vi "MS SQL_Count_RFID_STN10.vi"(8 "error in (no error)":errorcluster, 11 "Ref in":T1={"MS SQL Connection"=refnum, "UDL File"=path "", "Time"="", "DCODE"="", "WIP+1"=0, "MC No?"=0, "POKAYOKE?"=FALSE, "Expected Result"="", "Result [Status]"="", "Clock"=0.0, "RFID"="", "WIP Queue"=refnum, "TS Parameter"={"ProfitCenterCode"="", "LineCode"="", "WorkOrderNumber"="", "Model"="", "Model_with_Prefix"="", "VendorCode"="", "SetParameterDateCode"="", "PokaYoke"=0, "Target"=1, "Live_DateCode"="", "CustomerPartNumber"="", "Hand"="", "sBarcode"=FALSE, "FCA"=0, "Ent_Stamp"=timestamp(0 s since 1904-01-01), "STS_CD"=0.0}, "Data_Queue"=[], "RFID Serial No."=""} {"TS Parameter"."FCA" format="%01d"; "TS Parameter"."Target" min=1 max=100000; "TS Parameter"."PokaYoke" min=0 max=1}) -> (0 "error out":errorcluster, 1 "Count":i32 format="%02d", 2 "Count[s]":string, 3 "Ref Out":T1={"MS SQL Connection"=refnum, "UDL File"=path "", "Time"="", "DCODE"="", "WIP+1"=0, "MC No?"=0, "POKAYOKE?"=FALSE, "Expected Result"="", "Result [Status]"="", "Clock"=0.0, "RFID"="", "WIP Queue"=refnum, "TS Parameter"={"ProfitCenterCode"="", "LineCode"="", "WorkOrderNumber"="", "Model"="", "Model_with_Prefix"="", "VendorCode"="", "SetParameterDateCode"="", "PokaYoke"=0, "Target"=1, "Live_DateCode"="", "CustomerPartNumber"="", "Hand"="", "sBarcode"=FALSE, "FCA"=0, "Ent_Stamp"=timestamp(0 s since 1904-01-01), "STS_CD"=0.0}, "Data_Queue"=[], "RFID Serial No."=""} {"TS Parameter"."FCA" format="%01d"; "TS Parameter"."Target" min=1 max=100000; "TS Parameter"."PokaYoke" min=0 max=1}, 4 "resulting string":string)   [LabVIEW 2020]
uses:
  Controls/TD SQL.ctl
  <vilib>/addons/database/Connection.llb/Conn ObjectReference.ctl
  Controls/WIP_State.ctl
  Controls/TS_Parameter.ctl
  <vilib>/addons/database/Connection.llb/Conn Execute.vi
  <vilib>/addons/database/Recordset.llb/Rec Fetch Recordset Data (R).vi
  <vilib>/addons/database/Recordset.llb/Rec Destroy - Connection.vi
  <vilib>/addons/database/NI_Database_API.lvlib
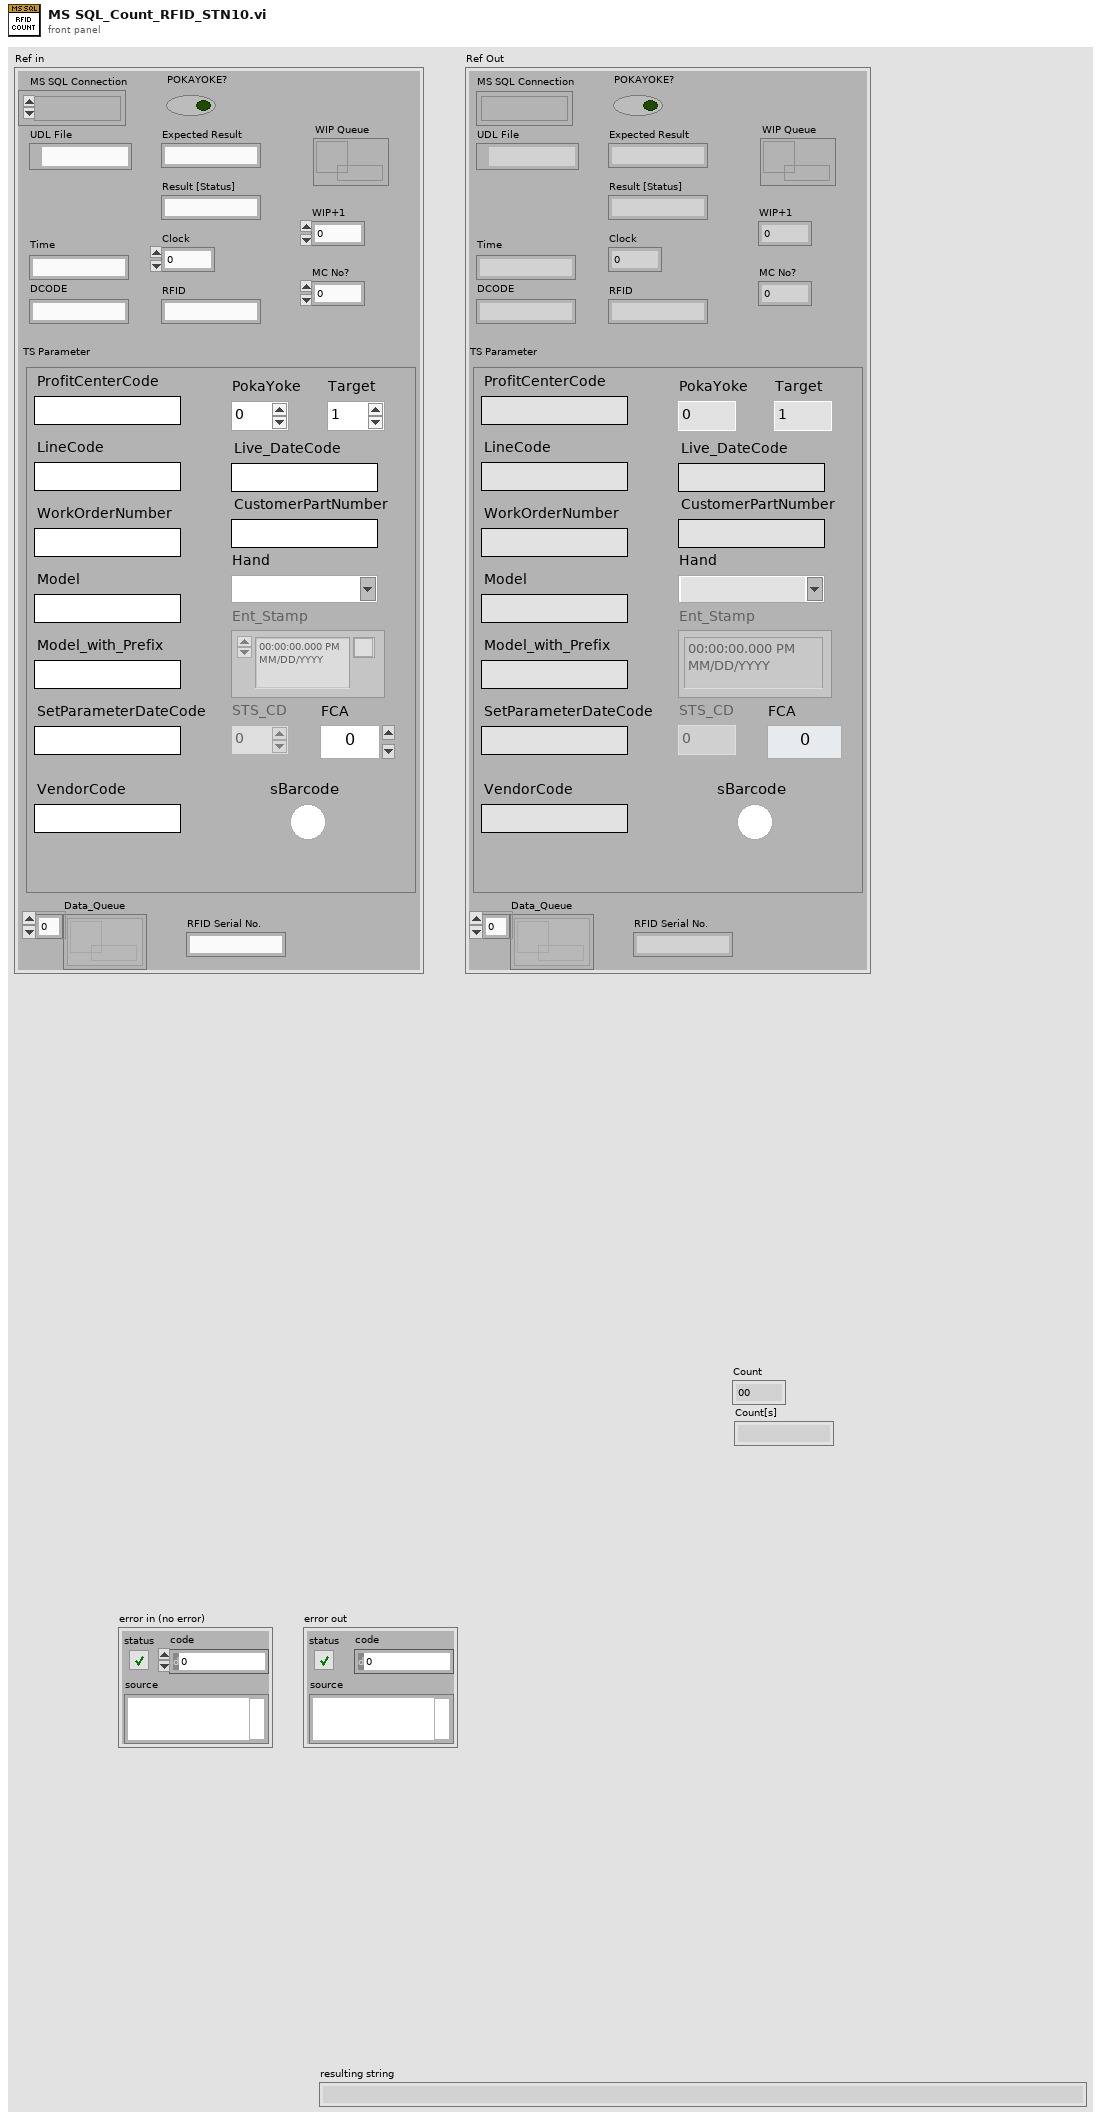
[diagram p1: front panel]
types:
  T1 = typedef "TD SQL.ctl" = cluster{"MS SQL Connection":T2, "UDL File":path, "Time":string, "DCODE":string, "WIP+1":i64, "MC No?":i32, "POKAYOKE?":bool, "Expected Result":string, "Result [Status]":string, "Clock":dbl, "RFID":string, "WIP Queue":refnum<queue>, "TS Parameter":T3, "Data_Queue":refnum<queue>[], "RFID Serial No.":string}
  T2 = typedef "NI_Database_API.lvlib/Conn ObjectReference.ctl" = refnum<k1>
  T3 = typedef "TS_Parameter.ctl" = cluster{"ProfitCenterCode":string, "LineCode":string, "WorkOrderNumber":string, "Model":string, "Model_with_Prefix":string, "VendorCode":string, "SetParameterDateCode":string, "PokaYoke":i32, "Target":i32, "Live_DateCode":string, "CustomerPartNumber":string, "Hand":string, "sBarcode":bool, "FCA":i32, "Ent_Stamp":timestamp, "STS_CD":dbl}
  T4 = typedef "NI_Database_API.lvlib/Rec ObjectReference.ctl" = refnum<k1>
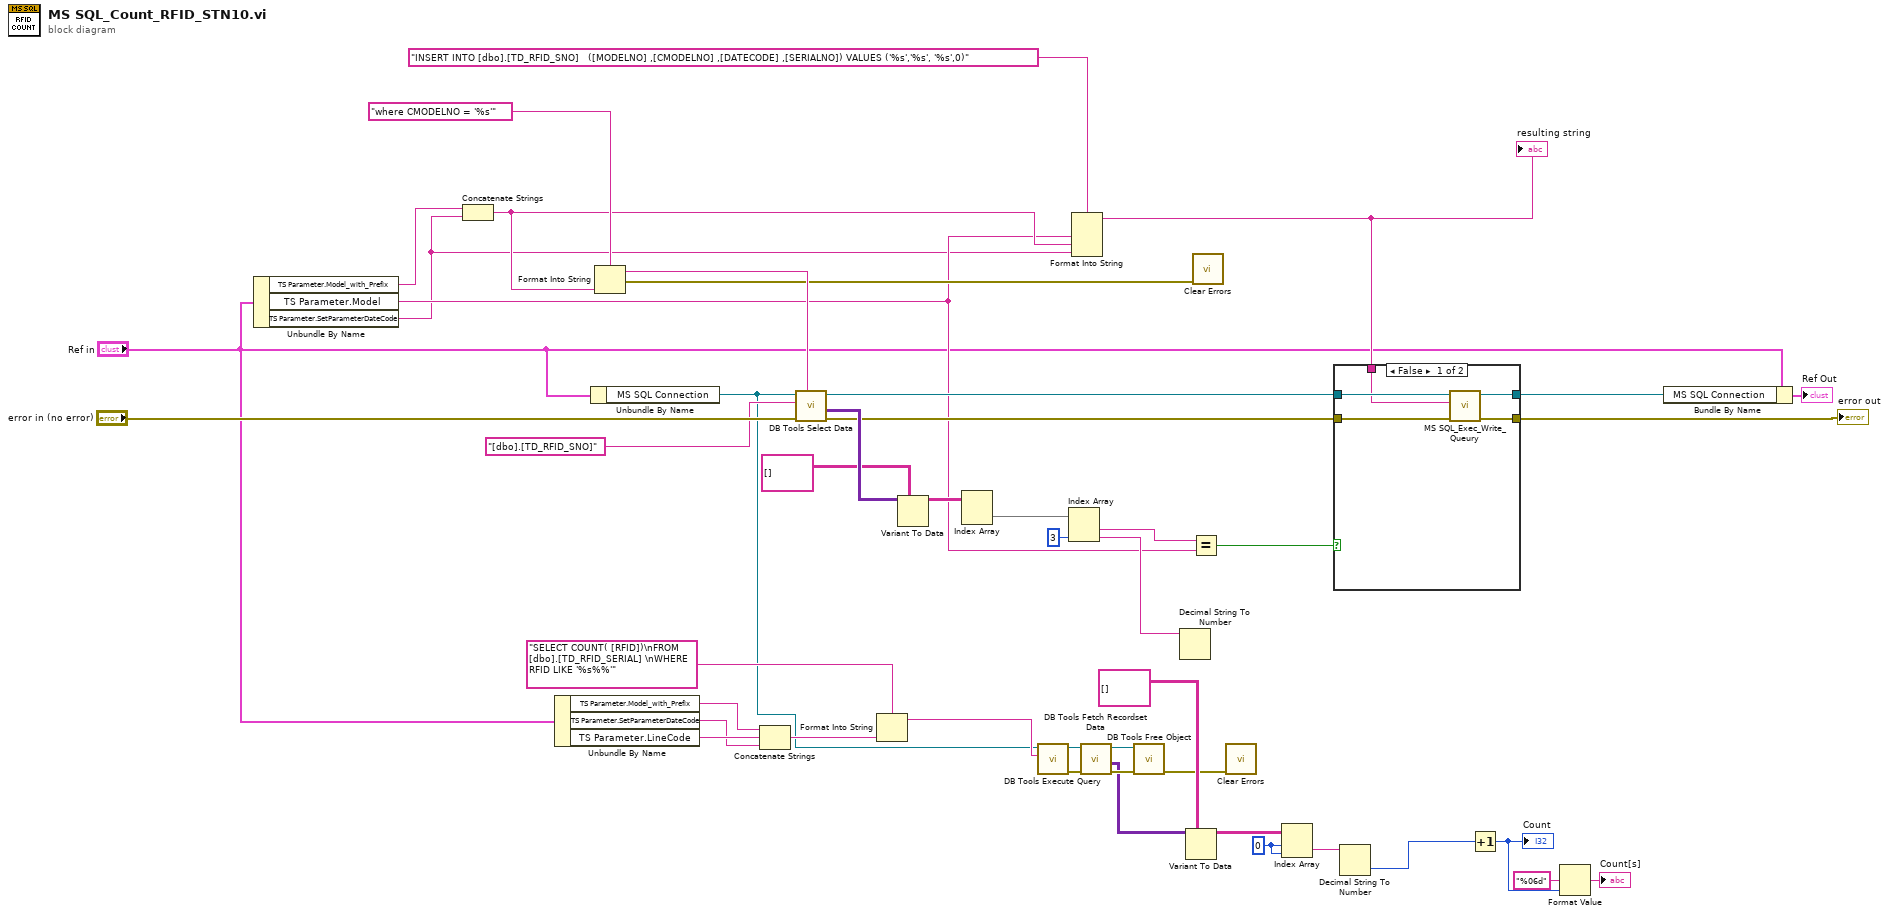
[diagram p0: block diagram]
diagram:
  w6 = 0 ("index (row)")
  n1 = Unbundle By Name("Ref in") -> ("TS Parameter.Model_with_Prefix"=w23:string, "TS Parameter.Model"=w21:string, "TS Parameter.SetParameterDateCode"=w20:string)
  n2 = Concatenate Strings(w23, w20) -> (w22:string)
  n3 = Unbundle By Name("Ref in") -> ("TS Parameter.Model_with_Prefix"=w18:string, "TS Parameter.SetParameterDateCode"=w16:string, "TS Parameter.LineCode"=w17:string)
  n4 = Unbundle By Name("Ref in") -> ("MS SQL Connection"=w2:T2)
  n5 = Format Into String(format string="where CMODELNO = '%s'", w22) -> (resulting string=w40:string, error out=w37:errorcluster)  [unwired: 2 in]
  n6 = Concatenate Strings(w18, w17, w16) -> (w15:string)
  n7 = call <vilib>:"DB Tools Select Data.vi"("condition"=w40, "error in (no error)"="error in (no error)", "table"="[dbo].[TD_RFID_SNO]", "connection reference"=w2) -> ("error out"=w32:errorcluster, "data"=w39:variant[][], "connection reference out"=w34:T2)  [unwired: 2 in]
  n8 = Format Into String(format string="SELECT COUNT( [RFID])\nFROM [dbo].[TD_RFID_SERIAL] \nWHERE RFID LIKE '%s%%'", w15) -> (resulting string=w4:string)  [unwired: 2 in, 1 out]
  n9 = Variant To Data(type=string[][] [] ("Data"), Variant=w39) -> (data=w36:string[][])  [unwired: 1 in, 1 out]
  n10 = Index Array(array=w36) -> (element=w35:string[])  [unwired: 2 in]
  n11 = call-poly <vilib>:"DB Tools Execute Query.vi"("SQL query"=w4, "connection reference"=w2) -> ("error out"=w12:errorcluster, "recordset reference"=w13:T4)  [unwired: 6 in]
  n12 = Index Array(array=w35, index #2=3 ("index")) -> (element #1=w30:string, element #2=w25:string)  [unwired: 1 in]
  n13 = Format Into String(format string="INSERT INTO [dbo].[TD_RFID_SNO]   ([MODELNO] ,[CMODELNO] ,[DATECODE] ,[SERIALNO]) VALUES ('%s','%s', '%s',0)" ("Query"), w21, w22, w20) -> (resulting string=w27:string)  [unwired: 2 in, 1 out]
  "resulting string" <- w27
  n14 = call-poly <vilib>:"DB Tools Fetch Recordset Data.vi"("error in (no error)"=w12, "recordset reference"=w13) -> ("error out"=w11:errorcluster, "recordset data"=w10:variant[][], "recordset reference out"=w14:T4)  [unwired: 3 in]
  n15 = call-poly <vilib>:"DB Tools Free Object.vi"("error in (no error)"=w11, "recordset reference"=w14) -> ("error out"=w8:errorcluster)  [unwired: 8 in, 1 out]
  n16 = Decimal String To Number(string=w25) -> ()  [unwired: 2 in, 2 out]
  n17 = Variant To Data(type=string[][] [] ("Data"), Variant=w10) -> (data=w7:string[][])  [unwired: 1 in, 1 out]
  n18 = Equal?(x=w30, y=w21) -> (x = y?=w29:bool)
  n19 = call <vilib>:"Clear Errors.vi"("error in (no error)"=w37) -> ()  [unwired: 5 in, 2 out]
  n20 = call <vilib>:"Clear Errors.vi"("error in (no error)"=w8) -> ()  [unwired: 5 in, 2 out]
  n21 = Index Array(array=w7, index (row)=w6, index (col)=w6) -> (element=w5:string)
  n22 = case shown="False" w29 {
    tunnel: w34 -> [w51 w53]
    tunnel: [w50 w53] -> w33
    tunnel: w32 -> [w49 w52]
    tunnel: [w48 w52] -> w31
    tunnel: w27 -> [w47 _]
    frame False {
      n23 = call "MS SQL_Exec_Write_Queury.vi"("error in (no error)"=w49, "Query"=w47, "Refnum in"=w51) -> ("error out"=w48:errorcluster, "Refnum out"=w50:T2)  [unwired: 7 in]
    }
    frame True {
    }
  }
  "error out" <- w31
  n24 = Decimal String To Number(string=w5) -> (number=w1:i32)  [unwired: 2 in, 1 out]
  n25 = Increment(x=w1) -> (x+1=w43:i32)
  "Count" <- w43
  n26 = Format Value(format string="%06d", value (0)=w43) -> (output string=→"Count[s]":string)  [unwired: 1 in]
  n27 = Bundle By Name(cluster="Ref in", "MS SQL Connection"=w33) -> (→"Ref Out":T1)
